vi "Write ROB info cluster element.vi"(7 "Update timestamp (F)":bool, 8 "error in (no error)":errorcluster, 9 "ROB Info-display":T1={"ID:"=-1, "State:"="UNKNOWN", "Voltages"=0, "Temp:"=-1.0, "Latch count:"=-1, "VRef:"=enum."Unknown", "Trigthres:"=0, "MPPC EN"=FALSE, "Test charge"=FALSE, "Responding"=FALSE, "Last update"=timestamp(0 s since 1904-01-01)} {"Last update" format="%<%X>T"; "Trigthres:" format="%.0fmV"; "Temp:" format="%.2f C"}, 10 "Channel":i32=-1, 11 "Hist cluster":T2) -> (0 "error out":errorcluster, 3 "Hist cluster":T2)   [LabVIEW 2016]
uses:
  Typedefs/All ROBs info cluster refnum.ctl
  Typedefs/ROB display info.ctl
panel:
  # "Leave channel unwired to use ROB info ID"
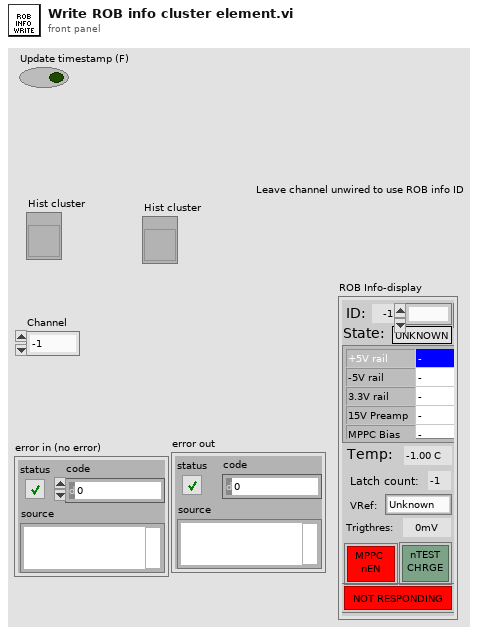
[diagram p1: front panel]
types:
  T1 = typedef "ROB display info.ctl" = cluster{"ID:":i32, "State:":string, "Voltages":i32, "Temp:":dbl, "Latch count:":i32, "VRef:":enum16{"External", "Internal", "Unknown"}, "Trigthres:":i32, "MPPC EN":bool, "Test charge":bool, "Responding":bool, "Last update":timestamp}
  T2 = typedef "All ROBs info cluster refnum.ctl" = refnum<vi>
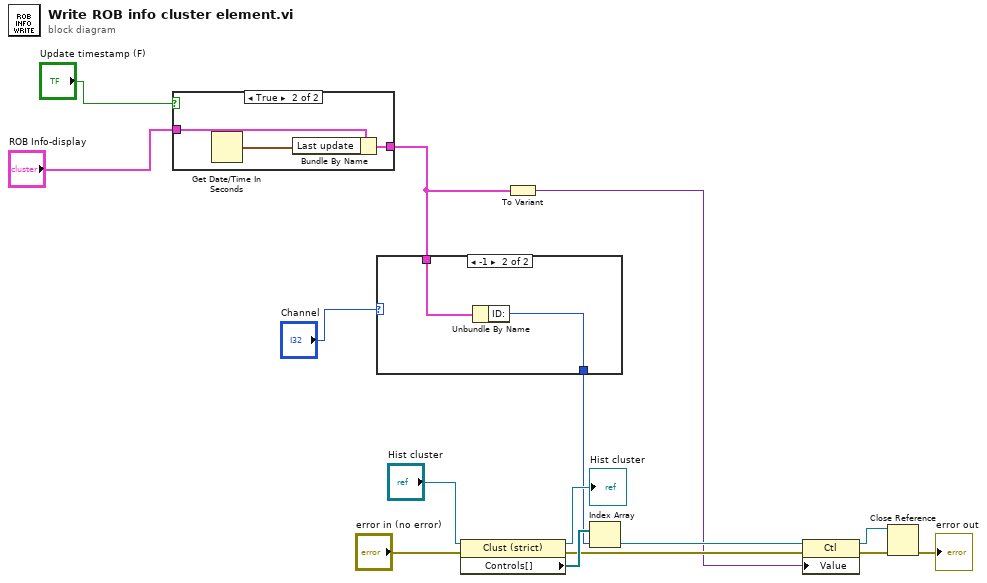
[diagram p0: block diagram]
diagram:
  n1 = case shown="True" "Update timestamp (F)" {
    tunnel: "ROB Info-display" -> [w16 w19]
    tunnel: [w16 w17] -> w1
    frame False {
    }
    frame True {
      n2 = Get Date/Time In Seconds() -> (seconds since 1Jan1904=w18:timestamp)
      n3 = Bundle By Name(cluster=w19, "Last update"=w18) -> (w17:T1)
    }
  }
  n4 = case shown="-1" "Channel" {
    selector: "Channel" -> [w20 _]
    tunnel: [w20 w21] -> w4
    tunnel: w1 -> [_ w22]
    frame Default {
    }
    frame -1 {
      n5 = Unbundle By Name(w22) -> ("ID:"=w21:i32)
    }
  }
  n6 = property class="Clust (strict)"(reference="Hist cluster", error in="error in (no error)") -> (reference out=→"Hist cluster":T2, error out=w12:errorcluster, "Controls[]"=w14:refnum<vi>[])
  n7 = To Variant(anything=w1) -> (Variant=w6:variant)
  n8 = Index Array(array=w14, index=w4) -> (element=w13:refnum<vi>)
  n9 = property class="Ctl"(reference=w13, error in=w12, "Value"=w6) -> (reference out=w8:refnum<vi>, error out=w9:errorcluster)
  n10 = Close Reference(reference=w8, error in (no error)=w9) -> (error out=→"error out":errorcluster)
